vi "Map to Locations.vi"(10 "Map in":bool[][](array[boolean])=[[FALSE, FALSE, FALSE, FALSE, FALSE, FALSE, TRUE, TRUE, FALSE, FALSE, FALSE, FALSE, FALSE], [FALSE, FALSE, FALSE, FALSE, FALSE, TRUE, TRUE, TRUE, TRUE, FALSE, FALSE, FALSE, FALSE], [FALSE, TRUE, FALSE, FALSE, FALSE, TRUE, FALSE, FALSE, TRUE, FALSE, FALSE, FALSE, TRUE], [FALSE, TRUE, TRUE, FALSE, FALSE, TRUE, FALSE, FALSE, TRUE, FALSE, FALSE, TRUE, TRUE], [FALSE, FALSE, TRUE, TRUE, FALSE, TRUE, FALSE, FALSE, TRUE, FALSE, TRUE, TRUE, FALSE], [FALSE, FALSE, FALSE, TRUE, TRUE, TRUE, FALSE, FALSE, TRUE, TRUE, TRUE, FALSE, FALSE], [FALSE, FALSE, FALSE, FALSE, TRUE, TRUE, TRUE, TRUE, TRUE, TRUE, FALSE, FALSE, FALSE], [FALSE, FALSE, FALSE, FALSE, FALSE, TRUE, FALSE, FALSE, TRUE, FALSE, FALSE, FALSE, FALSE], [FALSE, FALSE, FALSE, FALSE, FALSE, TRUE, FALSE, FALSE, TRUE, FALSE, FALSE, FALSE, FALSE]]) -> (2 "Locations":i32[][](array[numeric]))   [LabVIEW 2015]
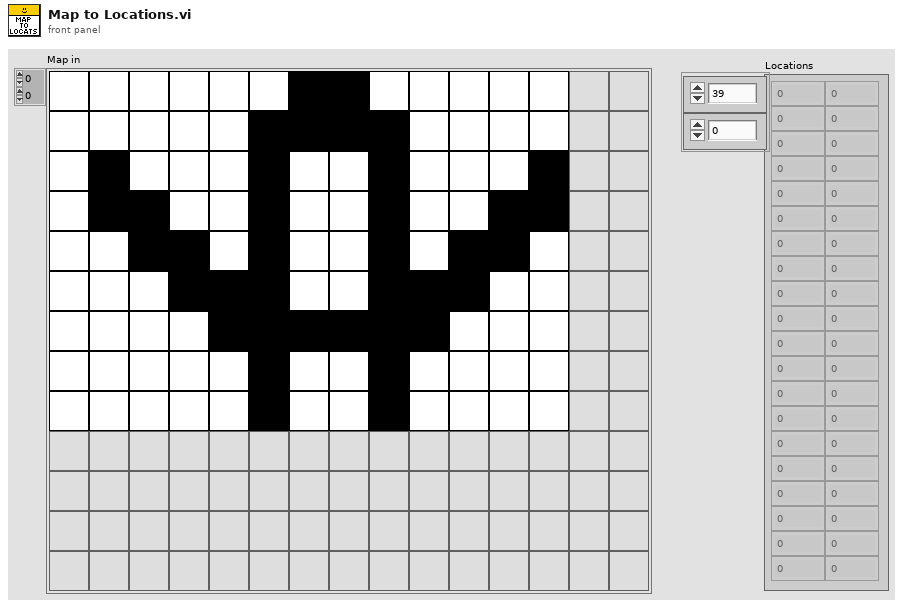
[diagram p1: front panel]
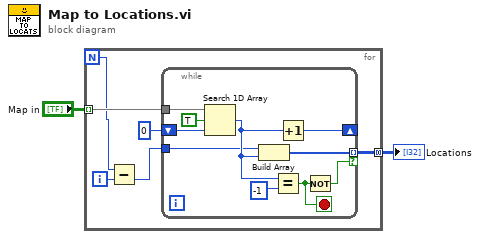
[diagram p0: block diagram]
diagram:
  n1 = for {
    N -> [w3]
    tunnel: "Map in" -> [w8] mode=indexing
    tunnel: [w7] -> w2 mode=concatenating
    i -> [w5]
    n2 = Subtract(x=w3, y=w5) -> (x-y=w4:i32)
    n3 = while {
      tunnel: w8 -> [w18]
      shift-right: [w11] -> _
      shift-left: 0 ("index of element") -> [w10]
      tunnel: w4 -> [w15]
      tunnel: [w14] -> w7 mode=indexing if=w12
      stop <- w13 stop-if-true
      n4 = Search 1D Array(1D array=w18, element=TRUE ("Element"), start index (0)=w10) -> (index of element=w16:i32)
      n5 = Build Array(w15, w16) -> (w14:i32[])
      n6 = Equal?(x=w16, y=-1) -> (x = y?=w13:bool)
      n7 = Increment(x=w16) -> (x+1=w11:i32)
      n8 = Not(x=w13) -> (.not. x?=w12:bool)
    }
  }
  "Locations" <- w2
